vi "XCtlExample.vi"() -> ()   [LabVIEW 2013]
uses:
  BarcodeType.ctl
  XControl/Barcode.xctl
  BarCodes.lvlib
panel:
  in  "Dark Color":u32(colorbox)
  in  "Light Color":u32(colorbox)=16777215
  in  "Scale":u8=2
  out "Barcode":string(xcontrol)
  in  "BarcodeType":T1
  in  "String":string="123456789012"
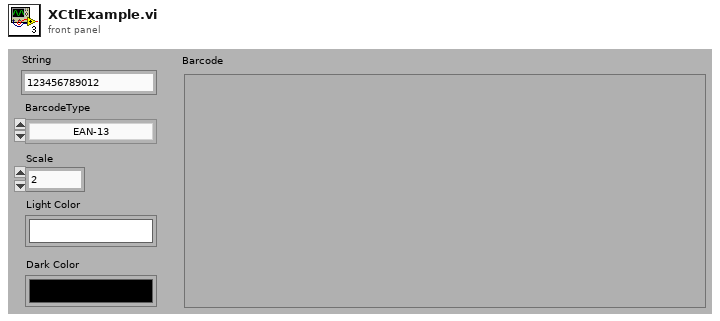
[diagram p1: front panel]
types:
  T1 = typedef "BarCodes.lvlib/BarcodeType.ctl" = enum16{"EAN-13", "UPC", "Code 39 (3 of 9)", "Code 128"}
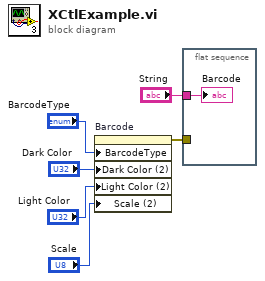
[diagram p0: block diagram]
diagram:
  n1 = property on="Barcode" class="Barcode (strict)"("BarcodeType"="BarcodeType", "Dark Color (2)"="Dark Color", "Light Color (2)"="Light Color", "Scale (2)"="Scale") -> (error out=w5:errorcluster)  [unwired: 2 in, 1 out]
  n2 = flat-sequence {
    tunnel: "String" -> [w7]
    tunnel: w5 -> [_]
    frame #0 {
      "Barcode" <- w7
    }
  }
